vi "Channel Array Size Error Test.vi"(8 "error in":errorcluster, 11 "NI 9474 test in":refnum<class "NI 9474 Test.lvclass">) -> (0 "error out":errorcluster, 3 "NI 9474 test out":refnum<class "NI 9474 Test.lvclass">)   [LabVIEW 2017, in "NI 9474 Test.lvclass"]
uses:
  NI 9474 Test.lvclass
  Module Test.lvclass
  Scripting/Modules/NI 9474/NI 9474.lvclass
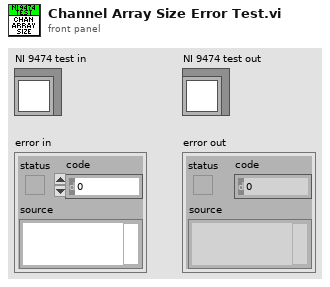
[diagram p1: front panel]
types:
  T1 = typedef "Scan Engine Scripting.lvlib/digital channel settings.ctl" = cluster{"name":string, "default value":bool}
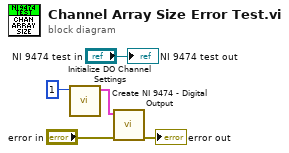
[diagram p0: block diagram]
diagram:
  n1 = call "Initialize DO Channel Settings.vi"("array size"=1) -> ("channel settings"=w4:T1[])  [unwired: 10 in]
  n2 = call "Create NI 9474 - Digital Output.vi"("error in"="error in", "channel settings"=w4) -> ("error out"=→"error out":errorcluster)  [unwired: 8 in, 1 out]
  "NI 9474 test out" <- "NI 9474 test in"
